vi "processPubDataPublish.vi"(8 "error in (no error)":errorcluster, 11 "MiddlewareSALThisComponent in":refnum<class "MiddlewareSALThisComponent.lvclass">) -> (0 "error out":errorcluster, 3 "MiddlewareSALThisComponent out":refnum<class "MiddlewareSALThisComponent.lvclass">)   [LabVIEW 2016, in "MiddlewareSALThisComponent.lvclass"]
uses:
  MiddlewareSALThisComponent.lvclass
  home/harini/tcs/ts_sedspectrometer/ComponentTemplateCore/ComponentModel/ComponentModel/Middleware/Middleware.lvclass
  ComponentTemplateCore/ComponentModel/ComponentModel/Middleware/Middleware.lvclass/Middleware.ctl
  ComponentTemplateCore/ComponentModel/ComponentModel/MiddlewareProcessEvent/MiddlewareProcessEvent.lvclass/MiddlewareProcessEvent.ctl
  MiddlewareSALThisComponent.lvclass/MiddlewareSALThisComponent.ctl
  PubSubDataEvent/PubSubDataEvent.lvclass/PubSubDataEvent.ctl
  <vilib>/Utility/error.llb/DialogType.ctl
  ts_sallv_sedspectrometer/DataTypes/logevent_ErrorCode.ctl
  ts_sallv_sedspectrometer/DataTypes/logevent_Heartbeat.ctl
  ts_sallv_sedspectrometer/DataTypes/LoopTime_ms.ctl
  ts_sallv_sedspectrometer/DataTypes/logevent_LoopTimeOutOfRange.ctl
  ts_sallv_sedspectrometer/DataTypes/logevent_RejectedCommand.ctl
  ts_sallv_sedspectrometer/DataTypes/logevent_SummaryState.ctl
  ts_sallv_sedspectrometer/DataTypes/Timestamp.ctl
  ts_sallv_sedspectrometer/DataTypes/logevent_DetailedState.ctl
  ts_sallv_sedspectrometer/DataTypes/logevent_AppliedSettingsMatchStart.ctl
  ts_sallv_sedspectrometer/DataTypes/logevent_SettingVersions.ctl
  ts_sallv_sedspectrometer/DataTypes/logevent_MeasuredSpectrum.ctl
  ts_sallv_sedspectrometer/DataTypes/logevent_Timeout.ctl
  ComponentTemplateCore/ComponentModel/ComponentModel/Middleware/Middleware.lvclass
  ComponentTemplateCore/ComponentModel/ComponentModel/MiddlewareProcessEvent/MiddlewareProcessEvent.lvclass
  PubSubDataEvent/PubSubDataEvent.lvclass
  ts_sallv_sedspectrometer/SALLV_sedSpectrometer.lvlib
  ProgrammaticInitialization/ProgrammaticInitialization.lvclass
panel:
  out "disconnect":bool
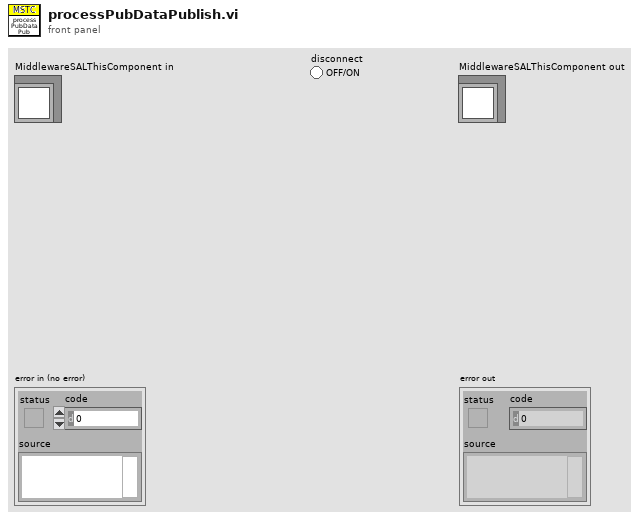
[diagram p1: front panel]
types:
  T1 = typedef "TypedefsDataEvents.lvlib/PubDataEvents.ctl" = cluster{"AppliedSettingsMatchStart":refnum<user-event>, "SettingVersions":refnum<user-event>, "SummaryState":refnum<user-event>, "RejectedCommand":refnum<user-event>, "DetailedState":refnum<user-event>, "ErrorCode":refnum<user-event>, "Heartbeat":refnum<user-event>, "LoopTime_ms":refnum<user-event>, "LoopTimeOutOfRange":refnum<user-event>, "Timestamp":refnum<user-event>, "TimeOut":refnum<user-event>, "MeasuredSpectrum":refnum<user-event>}
  T2 = typedef "MiddlewareProcessEvents.ctl" = cluster{"disconnect":refnum<user-event>, "error":refnum<user-event>}
  T3 = typedef "SALLV_sedSpectrometer.lvlib/logevent_ErrorCode.ctl" = cluster{"errorCode":i32, "priority":i32}
  T4 = typedef "SALLV_sedSpectrometer.lvlib/logevent_Heartbeat.ctl" = cluster{"heartbeat":bool, "priority":i32}
  T5 = typedef "SALLV_sedSpectrometer.lvlib/LoopTime_ms.ctl" = cluster{"loopTime_ms":dbl}
  T6 = typedef "SALLV_sedSpectrometer.lvlib/logevent_LoopTimeOutOfRange.ctl" = cluster{"loopTimeOutOfRange":bool, "priority":i32}
  T7 = typedef "SALLV_sedSpectrometer.lvlib/logevent_RejectedCommand.ctl" = cluster{"commandValue":u16, "detailedState":u16, "timestamp":dbl, "priority":i32}
  T8 = typedef "SALLV_sedSpectrometer.lvlib/logevent_SummaryState.ctl" = cluster{"summaryState":enum32{"", "DisabledState", "EnabledState", "FaultState", "OfflineState", "StandbyState"}, "priority":i32}
  T9 = typedef "SALLV_sedSpectrometer.lvlib/Timestamp.ctl" = cluster{"timestamp":dbl}
  T10 = typedef "SALLV_sedSpectrometer.lvlib/logevent_DetailedState.ctl" = cluster{"detailedState":enum32{"", "DisabledState", "EnabledState", "FaultState", "OfflineState", "StandbyState", "CaptureSpectImage", "NotImaging"}, "priority":i32}
  T11 = typedef "SALLV_sedSpectrometer.lvlib/logevent_AppliedSettingsMatchStart.ctl" = cluster{"appliedSettingsMatchStartIsTrue":bool, "priority":i32}
  T12 = typedef "SALLV_sedSpectrometer.lvlib/logevent_SettingVersions.ctl" = cluster{"recommendedSettingsVersion":string, "recommendedSettingsLabels":string, "priority":i32}
  T13 = typedef "SALLV_sedSpectrometer.lvlib/logevent_MeasuredSpectrum.ctl" = cluster{"imageName":string, "wavelength[2048]":dbl[], "intensity[2048]":dbl[], "integrationTime":sgl, "temperature":dbl, "priority":i32}
  T14 = typedef "SALLV_sedSpectrometer.lvlib/logevent_Timeout.ctl" = cluster{"timeout":bool, "priority":i32}
  T15 = typedef "DialogType.ctl" = u16
  T16 = enum32{"", "DisabledState", "EnabledState", "FaultState", "OfflineState", "StandbyState"}
  T17 = typedef "SEDSpectrometerTypedefs.lvlib/CommandValue.ctl" = enum16{"clearError", "disable", "enable", "exit", "GoToStandby", "OnHeartbeat", "OnIncomingMessagingError", "OnInterrupt", "start", "captureSpectImage", "setSpectTempSetpoint", "stopImageCapture"}
  T18 = enum32{"", "DisabledState", "EnabledState", "FaultState", "OfflineState", "StandbyState", "CaptureSpectImage", "NotImaging"}
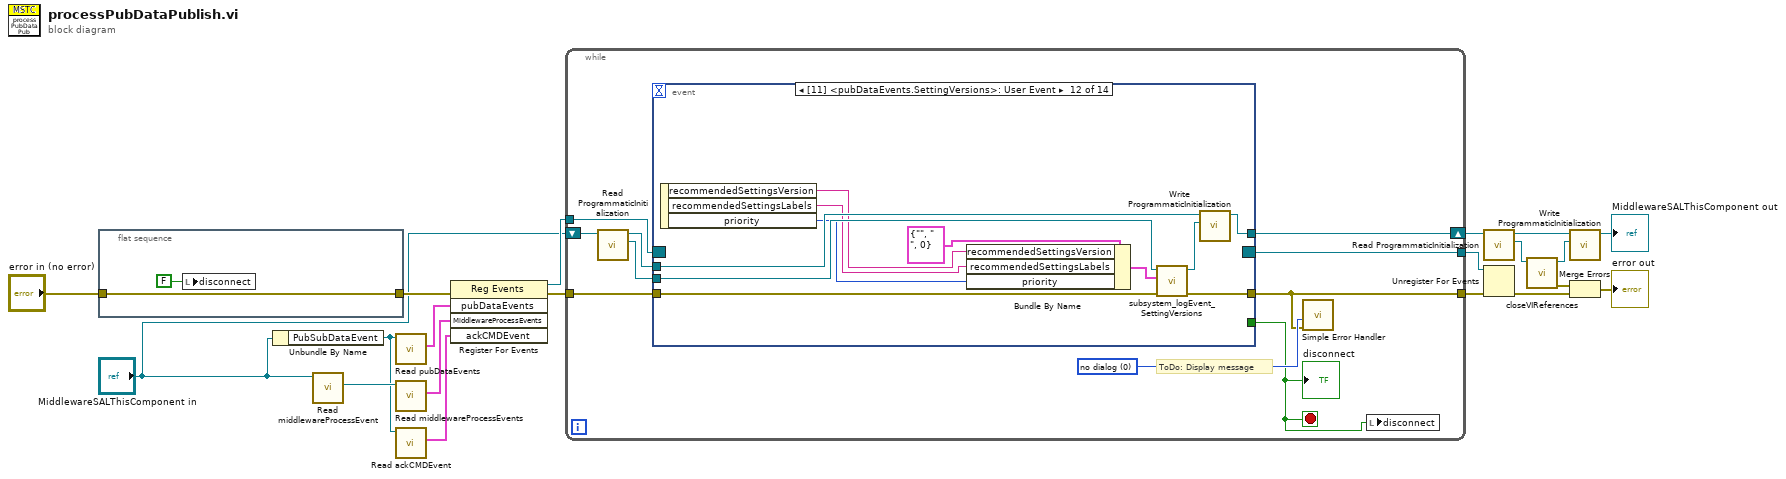
[diagram p0: block diagram]
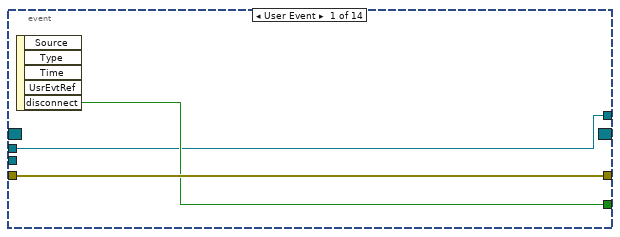
[diagram p2: hidden frame]
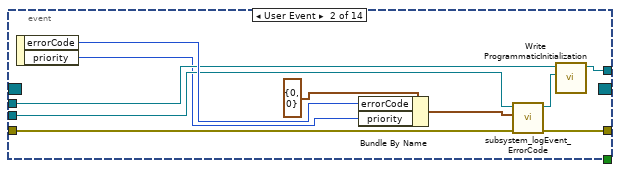
[diagram p3: hidden frame]
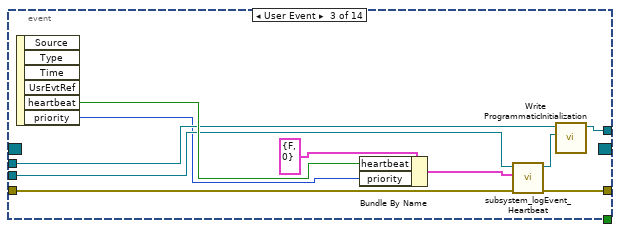
[diagram p4: hidden frame]
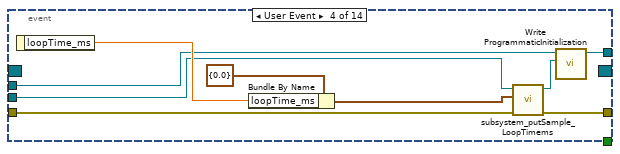
[diagram p5: hidden frame]
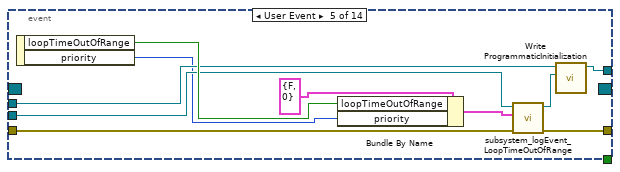
[diagram p6: hidden frame]
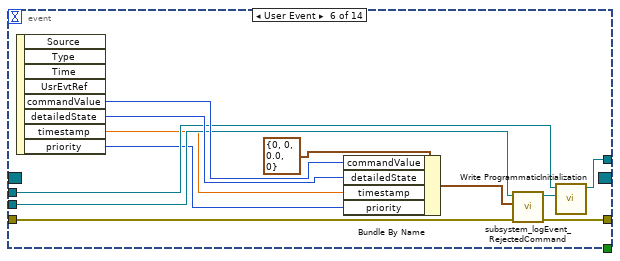
[diagram p7: hidden frame]
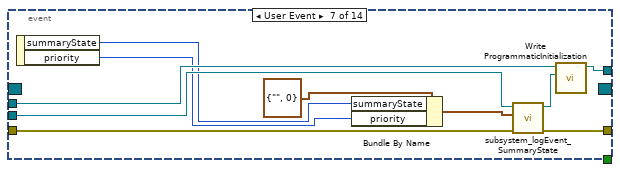
[diagram p8: hidden frame]
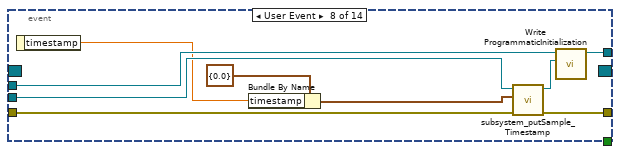
[diagram p9: hidden frame]
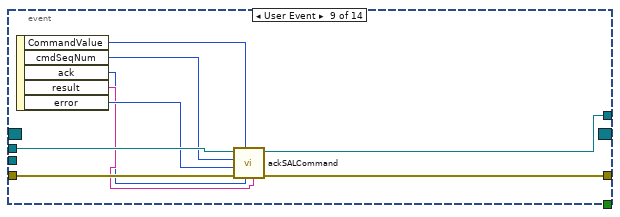
[diagram p10: hidden frame]
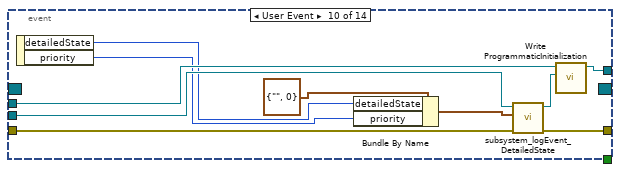
[diagram p11: hidden frame]
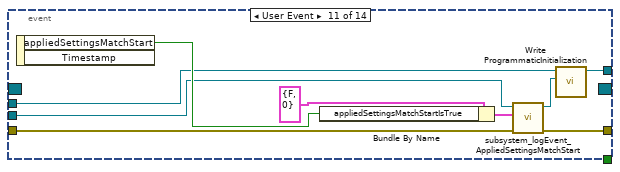
[diagram p12: hidden frame]
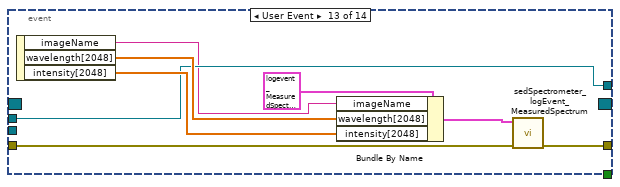
[diagram p13: hidden frame]
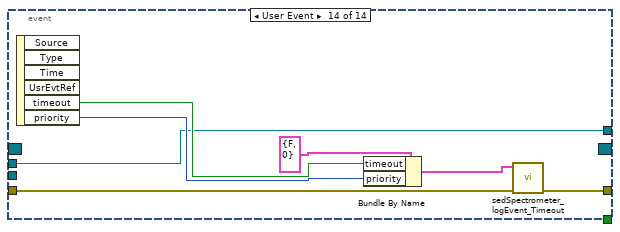
[diagram p14: hidden frame]
diagram:
  n1 = flat-sequence {
    tunnel: [w22] -> w16
    tunnel: "error in (no error)" -> [w22]
    frame #0 {
      n2 = local write "disconnect"(FALSE ("disconnect")) -> ()
    }
  }
  n3 = Unbundle By Name("MiddlewareSALThisComponent in") -> ("PubSubDataEvent"=w12:refnum<class "PubSubDataEvent.lvclass">)
  n4 = call "Read middlewareProcessEvent.vi"("Middleware in"="MiddlewareSALThisComponent in") -> ("middlewareProcessEvent"=w20:refnum<class "MiddlewareProcessEvent.lvclass">)  [unwired: 9 in, 1 out]
  n5 = call "Read pubDataEvents.vi"("PubSubDataEvent in"=w12) -> ("pubDataEvents"=w15:T1)  [unwired: 9 in, 1 out]
  n6 = call "Read middlewareProcessEvents.vi"("MiddlewareProcessEvent in"=w20) -> ("MiddlewareProcessEvents"=w11:T2)  [unwired: 9 in, 1 out]
  n7 = call "Read ackCMDEvent.vi"("PubSubDataEvent in"=w12) -> ("ackCMDEvent"=w10:cluster{"ackCMD":refnum<user-event>})  [unwired: 8 in, 2 out]
  n8 = register-events(error in=w16, w15, w11, w10) -> (reference out=w19:refnum<event-registration>, error out=w18:errorcluster)  [unwired: 1 in]
  n9 = while {
    tunnel: w19 -> [w32]
    tunnel: [w30] -> w13
    tunnel: w18 -> [w29]
    tunnel: [w28] -> w14
    shift-right: [w26] -> w5
    shift-left: "MiddlewareSALThisComponent in" -> [w24]
    stop <- w27 stop-if-true
    w31 = T15 0 items=["no dialog", "OK message", "continue or stop message", "OK message + warnings", "continue/stop + warnings"] ("type of dialog (OK msg:1)")
    # "ToDo: Display message"
    n10 = call-dynamic "Read ProgrammaticInitialization.vi"("MiddlewareSALThisComponent in"=w24) -> ("ProgrammaticInitialization"=w25:refnum<class "ProgrammaticInitialization.lvclass">, "MiddlewareSALThisComponent out"=w23:refnum<class "MiddlewareSALThisComponent.lvclass">)  [unwired: 8 in, 1 out]
    n11 = event shown="[11] <pubDataEvents.SettingVersions>: User Event" {
      selector: w32 -> [_ _ _ _ _ _ _ _ _ _ _ _ _ _]
      dyn-events: [_ _ _ _ _ _ _ _ _ _ _ _ _ _] -> w28
      timeout: _ -> [_ _ _ _ _ _ _ _ _ _ _ _ _ _]
      tunnel: [w34 _ _ _ _ _ _ _ _ _ _ _ _ _] -> w27
      tunnel: [w35 w43 w53 w62 w72 w83 w95 w104 w106 w123 w130 w143 w147 w154] -> w30
      tunnel: w29 -> [w35 w37 w52 w61 w71 w77 w94 w97 w113 w122 w125 w138 w148 w159]
      tunnel: w23 -> [w33 w40 w49 w58 w68 w80 w91 w102 w114 w119 w129 w142 w146 w153]
      tunnel: [w33 w39 w48 w57 w67 w79 w90 w101 w107 w118 w127 w141 w146 w153] -> w26
      tunnel: w25 -> [_ w38 w50 w59 w69 w78 w92 w99 _ w120 w126 w139 _ _]
      event User Event {
        n12 = event-data() -> ("disconnect"=w34:bool)  [unwired: 1 in, 4 out]
      }
      event User Event {
        n13 = event-data() -> ("errorCode"=w44:i32, "priority"=w36:i32)  [unwired: 1 in]
        n14 = Bundle By Name(cluster=T3 {"errorCode"=0, "priority"=0} ("logevent_ErrorCode_Ctl"), "errorCode"=w44, "priority"=w36) -> (w42:T3)
        n15 = call "subsystem_logEvent_ErrorCode.vi"("error in (no error)"=w37, "logevent_ErrorCode in"=w42, "ProgrammaticInitialization in"=w38) -> ("error out"=w43:errorcluster, "ProgrammaticInitialization out"=w41:refnum<class "ProgrammaticInitialization.lvclass">)  [unwired: 6 in, 1 out]
        n16 = call-dynamic "Write ProgrammaticInitialization.vi"("ProgrammaticInitialization"=w41, "MiddlewareSALThisComponent in"=w40) -> ("MiddlewareSALThisComponent out"=w39:refnum<class "MiddlewareSALThisComponent.lvclass">)  [unwired: 8 in, 1 out]
      }
      event User Event {
        n17 = event-data() -> ("heartbeat"=w55:bool, "priority"=w46:i32)  [unwired: 1 in, 4 out]
        n18 = Bundle By Name(cluster=T4 {"heartbeat"=FALSE, "priority"=0} ("logevent_Heartbeat_Ctl"), "heartbeat"=w55, "priority"=w46) -> (w51:T4)
        n19 = call "subsystem_logEvent_Heartbeat.vi"("error in (no error)"=w52, "logevent_Heartbeat in"=w51, "ProgrammaticInitialization in"=w50) -> ("error out"=w53:errorcluster, "ProgrammaticInitialization out"=w47:refnum<class "ProgrammaticInitialization.lvclass">)  [unwired: 6 in, 1 out]
        n20 = call-dynamic "Write ProgrammaticInitialization.vi"("ProgrammaticInitialization"=w47, "MiddlewareSALThisComponent in"=w49) -> ("MiddlewareSALThisComponent out"=w48:refnum<class "MiddlewareSALThisComponent.lvclass">)  [unwired: 8 in, 1 out]
      }
      event User Event {
        n21 = event-data() -> ("loopTime_ms"=w63:dbl)  [unwired: 1 in]
        n22 = Bundle By Name(cluster=T5 {"loopTime_ms"=0.0} ("LoopTime_ms_Ctl"), "loopTime_ms"=w63) -> (w60:T5)
        n23 = call "subsystem_putSample_LoopTimems.vi"("error in (no error)"=w61, "LoopTime_ms in"=w60, "ProgrammaticInitialization in"=w59) -> ("error out"=w62:errorcluster, "ProgrammaticInitialization out"=w56:refnum<class "ProgrammaticInitialization.lvclass">)  [unwired: 6 in, 1 out]
        n24 = call-dynamic "Write ProgrammaticInitialization.vi"("ProgrammaticInitialization"=w56, "MiddlewareSALThisComponent in"=w58) -> ("MiddlewareSALThisComponent out"=w57:refnum<class "MiddlewareSALThisComponent.lvclass">)  [unwired: 8 in, 1 out]
      }
      event User Event {
        n25 = event-data() -> ("loopTimeOutOfRange"=w73:bool, "priority"=w65:i32)  [unwired: 1 in]
        n26 = Bundle By Name(cluster=T6 {"loopTimeOutOfRange"=FALSE, "priority"=0} ("logevent_LoopTimeOutOfRange_Ctl"), "loopTimeOutOfRange"=w73, "priority"=w65) -> (w70:T6)
        n27 = call "subsystem_logEvent_LoopTimeOutOfRange.vi"("error in (no error)"=w71, "logevent_LoopTimeOutOfRange in"=w70, "ProgrammaticInitialization in"=w69) -> ("error out"=w72:errorcluster, "ProgrammaticInitialization out"=w66:refnum<class "ProgrammaticInitialization.lvclass">)  [unwired: 6 in, 1 out]
        n28 = call-dynamic "Write ProgrammaticInitialization.vi"("ProgrammaticInitialization"=w66, "MiddlewareSALThisComponent in"=w68) -> ("MiddlewareSALThisComponent out"=w67:refnum<class "MiddlewareSALThisComponent.lvclass">)  [unwired: 8 in, 1 out]
      }
      event User Event {
        n29 = event-data() -> ("commandValue"=w85:u16, "detailedState"=w84:u16, "timestamp"=w76:dbl, "priority"=w75:i32)  [unwired: 1 in, 4 out]
        n30 = Bundle By Name(cluster=T7 {"commandValue"=0, "detailedState"=0, "timestamp"=0.0, "priority"=0} ("logevent_RejectedCommand_Ctl"), "commandValue"=w85, "detailedState"=w84, "timestamp"=w76, "priority"=w75) -> (w82:T7)
        n31 = call "subsystem_logEvent_RejectedCommand.vi"("error in (no error)"=w77, "logevent_RejectedCommand in"=w82, "ProgrammaticInitialization in"=w78) -> ("error out"=w83:errorcluster, "ProgrammaticInitialization out"=w81:refnum<class "ProgrammaticInitialization.lvclass">)  [unwired: 6 in, 1 out]
        n32 = call-dynamic "Write ProgrammaticInitialization.vi"("ProgrammaticInitialization"=w81, "MiddlewareSALThisComponent in"=w80) -> ("MiddlewareSALThisComponent out"=w79:refnum<class "MiddlewareSALThisComponent.lvclass">)  [unwired: 8 in, 1 out]
      }
      event User Event {
        n33 = event-data() -> ("summaryState"=w88:T16, "priority"=w87:i32)  [unwired: 1 in]
        n34 = Bundle By Name(cluster=T8 {"summaryState"=enum."", "priority"=0} ("logevent_SummaryState_Ctl"), "summaryState"=w88, "priority"=w87) -> (w93:T8)
        n35 = call "subsystem_logEvent_SummaryState.vi"("error in (no error)"=w94, "logevent_SummaryState in"=w93, "ProgrammaticInitialization in"=w92) -> ("error out"=w95:errorcluster, "ProgrammaticInitialization out"=w89:refnum<class "ProgrammaticInitialization.lvclass">)  [unwired: 6 in, 1 out]
        n36 = call-dynamic "Write ProgrammaticInitialization.vi"("ProgrammaticInitialization"=w89, "MiddlewareSALThisComponent in"=w91) -> ("MiddlewareSALThisComponent out"=w90:refnum<class "MiddlewareSALThisComponent.lvclass">)  [unwired: 8 in, 1 out]
      }
      event User Event {
        n37 = event-data() -> ("timestamp"=w98:dbl)  [unwired: 1 in]
        n38 = Bundle By Name(cluster=T9 {"timestamp"=0.0} ("Timestamp_Ctl"), "timestamp"=w98) -> (w103:T9)
        n39 = call "subsystem_putSample_Timestamp.vi"("error in (no error)"=w97, "Timestamp in"=w103, "ProgrammaticInitialization in"=w99) -> ("error out"=w104:errorcluster, "ProgrammaticInitialization out"=w100:refnum<class "ProgrammaticInitialization.lvclass">)  [unwired: 6 in, 1 out]
        n40 = call-dynamic "Write ProgrammaticInitialization.vi"("ProgrammaticInitialization"=w100, "MiddlewareSALThisComponent in"=w102) -> ("MiddlewareSALThisComponent out"=w101:refnum<class "MiddlewareSALThisComponent.lvclass">)  [unwired: 8 in, 1 out]
      }
      event User Event {
        n41 = event-data() -> ("CommandValue"=w108:T17, "cmdSeqNum"=w109:i32, "ack"=w110:i32, "result"=w111:string, "error"=w112:i32)  [unwired: 1 in]
        n42 = call "ackSALCommand.vi"("result"=w111, "ack"=w110, "CommandValue"=w108, "error in (no error)"=w113, "error"=w112, "cmdSeqNum"=w109, "MiddlewareSALThisComponent in"=w114) -> ("error out"=w106:errorcluster, "MiddlewareSALThisComponent out"=w107:refnum<class "MiddlewareSALThisComponent.lvclass">)  [unwired: 3 in]
      }
      event User Event {
        n43 = event-data() -> ("detailedState"=w116:T18, "priority"=w115:i32)  [unwired: 1 in]
        n44 = Bundle By Name(cluster=T10 {"detailedState"=enum."", "priority"=0} ("logevent_DetailedState_Ctl"), "detailedState"=w116, "priority"=w115) -> (w121:T10)
        n45 = call "subsystem_logEvent_DetailedState.vi"("error in (no error)"=w122, "logevent_DetailedState in"=w121, "ProgrammaticInitialization in"=w120) -> ("error out"=w123:errorcluster, "ProgrammaticInitialization out"=w117:refnum<class "ProgrammaticInitialization.lvclass">)  [unwired: 6 in, 1 out]
        n46 = call-dynamic "Write ProgrammaticInitialization.vi"("ProgrammaticInitialization"=w117, "MiddlewareSALThisComponent in"=w119) -> ("MiddlewareSALThisComponent out"=w118:refnum<class "MiddlewareSALThisComponent.lvclass">)  [unwired: 8 in, 1 out]
      }
      event User Event {
        n47 = event-data() -> ("appliedSettingsMatchStart"=w133:bool)  [unwired: 1 in, 1 out]
        n48 = Bundle By Name(cluster=T11 {"appliedSettingsMatchStartIsTrue"=FALSE, "priority"=0} ("logevent_AppliedSettingsMatchStart_Ctl"), "appliedSettingsMatchStartIsTrue"=w133) -> (w131:T11)
        n49 = call "subsystem_logEvent_AppliedSettingsMatchStart.vi"("error in (no error)"=w125, "logevent_AppliedSettingsMatchStart in"=w131, "ProgrammaticInitialization in"=w126) -> ("error out"=w130:errorcluster, "ProgrammaticInitialization out"=w128:refnum<class "ProgrammaticInitialization.lvclass">)  [unwired: 6 in, 1 out]
        n50 = call-dynamic "Write ProgrammaticInitialization.vi"("ProgrammaticInitialization"=w128, "MiddlewareSALThisComponent in"=w129) -> ("MiddlewareSALThisComponent out"=w127:refnum<class "MiddlewareSALThisComponent.lvclass">)  [unwired: 8 in, 1 out]
      }
      event User Event {
        n51 = event-data() -> ("recommendedSettingsVersion"=w135:string, "recommendedSettingsLabels"=w134:string, "priority"=w137:i32)  [unwired: 1 in]
        n52 = Bundle By Name(cluster=T12 {"recommendedSettingsVersion"="", "recommendedSettingsLabels"="                                                                                                                                                                                                                                                                ", "priority"=0} ("logevent_SettingVersions"), "recommendedSettingsVersion"=w135, "recommendedSettingsLabels"=w134, "priority"=w137) -> (w144:T12)
        n53 = call "subsystem_logEvent_SettingVersions.vi"("error in (no error)"=w138, "logevent_SettingVersions in"=w144, "ProgrammaticInitialization in"=w139) -> ("error out"=w143:errorcluster, "ProgrammaticInitialization out"=w140:refnum<class "ProgrammaticInitialization.lvclass">)  [unwired: 6 in, 1 out]
        n54 = call-dynamic "Write ProgrammaticInitialization.vi"("ProgrammaticInitialization"=w140, "MiddlewareSALThisComponent in"=w142) -> ("MiddlewareSALThisComponent out"=w141:refnum<class "MiddlewareSALThisComponent.lvclass">)  [unwired: 8 in, 1 out]
      }
      event User Event {
        n55 = event-data() -> ("imageName"=w145:string, "wavelength[2048]"=w151:dbl[], "intensity[2048]"=w150:dbl[])  [unwired: 1 in]
        n56 = Bundle By Name(cluster=T13 {"imageName"="", "wavelength[2048]"=array[2048 elements], "intensity[2048]"=array[2048 elements], "integrationTime"=0.0, "temperature"=0.0, "priority"=0} ("logevent_MeasuredSpectrum_Ctl"), "imageName"=w145, "wavelength[2048]"=w151, "intensity[2048]"=w150) -> (w149:T13)
        n57 = call "sedSpectrometer_logEvent_MeasuredSpectrum.vi"("error in (no error)"=w148, "logevent_MeasuredSpectrum_Ctl"=w149) -> ("error out"=w147:errorcluster)  [unwired: 7 in, 2 out]
      }
      event User Event {
        n58 = event-data() -> ("timeout"=w158:bool, "priority"=w157:i32)  [unwired: 1 in, 4 out]
        n59 = Bundle By Name(cluster=T14 {"timeout"=FALSE, "priority"=0} ("logevent_TimeOut_Ctl"), "timeout"=w158, "priority"=w157) -> (w155:T14)
        n60 = call "sedSpectrometer_logEvent_Timeout.vi"("error in (no error)"=w159, "logevent_Timeout_Ctl"=w155) -> ("error out"=w154:errorcluster)  [unwired: 7 in, 2 out]
      }
    }
    "disconnect" <- w27
    n61 = call <vilib>:"Simple Error Handler.vi"("type of dialog (OK msg:1)"=w31, "error in (no error)"=w30) -> ()  [unwired: 3 in, 5 out]
    n62 = local write "disconnect"(w27) -> ()
  }
  n63 = call-dynamic "Read ProgrammaticInitialization.vi"("MiddlewareSALThisComponent in"=w5) -> ("ProgrammaticInitialization"=w8:refnum<class "ProgrammaticInitialization.lvclass">, "MiddlewareSALThisComponent out"=w7:refnum<class "MiddlewareSALThisComponent.lvclass">)  [unwired: 8 in, 1 out]
  n64 = Unregister For Events(event registration refnum=w14, error in=w13) -> (error out=w2:errorcluster)
  n65 = call "closeVIReferences.vi"("ProgrammaticInitialization in"=w8) -> ("error out"=w3:errorcluster, "ProgrammaticInitialization out"=w6:refnum<class "ProgrammaticInitialization.lvclass">)  [unwired: 9 in]
  n66 = call-dynamic "Write ProgrammaticInitialization.vi"("ProgrammaticInitialization"=w6, "MiddlewareSALThisComponent in"=w7) -> ("MiddlewareSALThisComponent out"=→"MiddlewareSALThisComponent out":refnum<class "MiddlewareSALThisComponent.lvclass">)  [unwired: 8 in, 1 out]
  n67 = Merge Errors(w3, w2) -> (→"error out":errorcluster)
